vi "Get Array Value at Index - Boolean.vi"(6 "Return Default if Null? (T)":bool=TRUE, 8 "error in (no error)":errorcluster, 9 "Default Value if JSON Null":bool, 10 "Index":i32, 11 "JSON Tree In (JSON Array)":variant) -> (0 "error out":errorcluster, 1 "is JSON Null?":bool, 2 "Boolean Value":bool, 3 "JSON Tree Out Passthrough":variant)   [LabVIEW 2011, in "i3-json.lvlib"]
doc: "Use this template to build a VI to use as a subVI."
uses:
  i3-json.lvlib
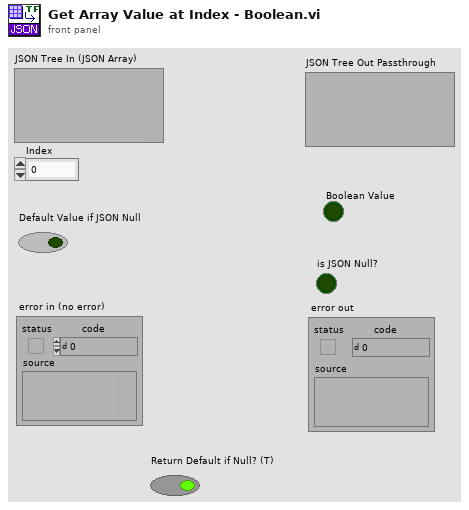
[diagram p1: front panel]
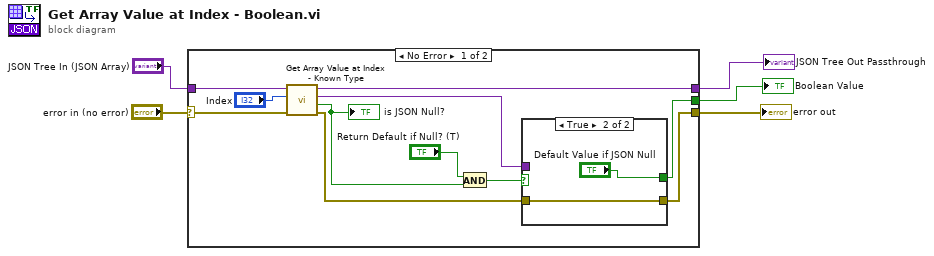
[diagram p0: block diagram]
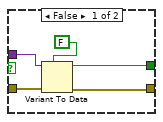
[diagram p2: hidden frame]
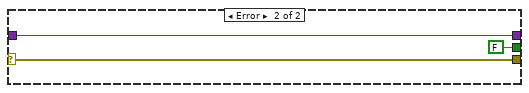
[diagram p3: hidden frame]
diagram:
  n1 = case shown="No Error" "error in (no error)" {
    selector: "error in (no error)" -> [w13 w26]
    tunnel: [w9 w26] -> w4
    tunnel: "JSON Tree In (JSON Array)" -> [w16 w25]
    tunnel: [w14 w25] -> w2
    tunnel: [w6 FALSE ("Default Value if JSON Null")] -> w1
    frame No Error {
      n2 = call "Get Array Value at Index - Known Type.vi"("error in (no error)"=w13, "Index"="Index", "JSON Tree In (JSON Array)"=w16) -> ("error out"=w10:errorcluster, "is JSON Null?"=w7:bool, "Value"=w8:variant, "JSON Tree Out Passthrough"=w14:variant)  [unwired: 3 in, 2 out]
      "is JSON Null?" <- w7
      n3 = And(x="Return Default if Null? (T)", y=w7) -> (x .and. y?=w11:bool)
      n4 = case shown="True" w11 {
        tunnel: w10 -> [w21 w23]
        tunnel: [w17 w23] -> w9
        tunnel: w8 -> [w20 _]
        tunnel: [w18 "Default Value if JSON Null"] -> w6
        frame False {
          n5 = Variant To Data(error in=w21, type=FALSE, Variant=w20) -> (data=w18:bool, error out=w17:errorcluster)
        }
        frame True {
        }
      }
    }
    frame Error {
    }
  }
  "error out" <- w4
  "JSON Tree Out Passthrough" <- w2
  "Boolean Value" <- w1
